vi "Update Time Msg.vi"(11 "Queue in":refnum<queue>) -> (3 "Queue out":refnum<queue>)   [LabVIEW 2018, in "Message Queue.lvlib"]
uses:
  Message Queue.lvlib
  Message Cluster.ctl
  Enqueue Message (Single).vi
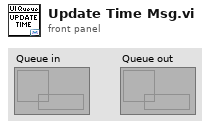
[diagram p1: front panel]
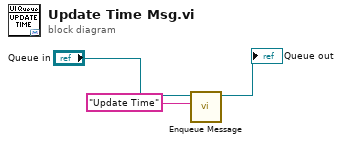
[diagram p0: block diagram]
diagram:
  n1 = call-poly "Enqueue Message.vi"("Message"="Update Time", "Message Queue"="Queue in") -> ("dup Message Queue"=→"Queue out":refnum<queue>)  [unwired: 8 in, 1 out]
